vi "HEAD.vi"(0 "client handle":T4, 1 "Error code options":T2={"1xx (info)"=FALSE, "2xx (success)"=FALSE, "3xx (redirect)"=FALSE, "4xx (client error)"=TRUE, "5xx (server error)"=TRUE, "Other"=TRUE}, 2 "BlueLogParent in":refnum<class "BlueLogParent_OpenSource.lvclass">, 5 "url":string, 11 "error in (no error)":errorcluster, 12 "timeout (10000)":i32=10000) -> (4 "client handle out":T4, 6 "headers":T3[](array[typedef]), 10 "HTTP response code":T1, 15 "error out":errorcluster)   [LabVIEW 2020, in "Blue Easy HTTP OpenSource.lvlib"]
doc: "Sends a Web request that returns headers from a server, Web page, or Web service. This VI uses the HEAD HTTP method. This VI does not submit any data to the server or receive body data. The minimal data exchange makes the HEAD VI useful for testing the validity of a URL. Refer to the World Wide Web Consortium Web site at www.w3.org for more information about HTTP method definitions, including the HEAD method.\n\nYou can assign a client handle to add authentication credentials, HTTP headers, or a cookie to Web requests made by the HEAD VI. Use the OpenHandle VI to open a client handle and establish credentials. Use the AddHeader VI to add header lines to Web requests made by the HEAD VI."
uses:
  Blue Easy HTTP OpenSource.lvlib
  <vilib>/httpClient/ClientHandle.ctl
  HTTP Header.ctl
  HTTP error on codes.ctl
  HTTP response code.ctl
  <userlib>/Blue Origin/BlueLogParent_OpenSource/BlueLogParentClass/BlueLogParent_OpenSource.lvclass
  Interpret Header.vi
  <vilib>/dlg_ctls.llb/Space Constant.vi
  <vilib>/Utility/error.llb/Trim Whitespace.vi
  <vilib>/Utility/error.llb/Error Cluster From Error Code.vi
  <vilib>/httpClient/LabVIEWHTTPClient.lvlib
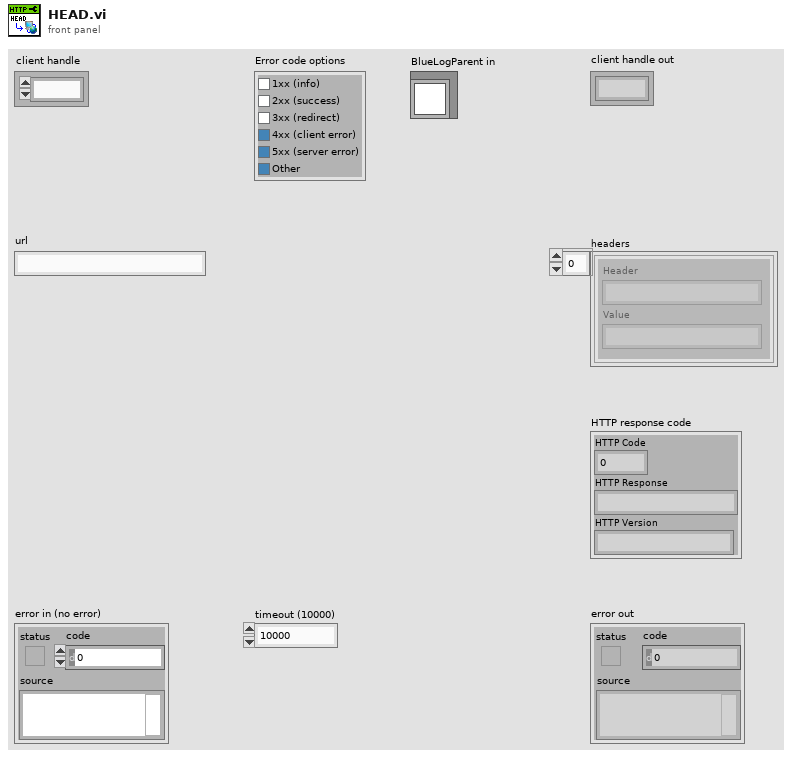
[diagram p1: front panel]
types:
  T1 = typedef "Blue Easy HTTP OpenSource.lvlib/HTTP response code.ctl" = cluster{"HTTP Code":u16, "HTTP Response":string, "HTTP Version":string}
  T2 = typedef "Blue Easy HTTP OpenSource.lvlib/HTTP error on codes.ctl" = cluster{"1xx (info)":bool, "2xx (success)":bool, "3xx (redirect)":bool, "4xx (client error)":bool, "5xx (server error)":bool, "Other":bool}
  T3 = typedef "Blue Easy HTTP OpenSource.lvlib/HTTP Header.ctl" = cluster{"Header":string, "Value":string}
  T4 = typedef "LabVIEWHTTPClient.lvlib/ClientHandle.ctl" = refnum<k1>
  T5 = typedef "BlueLogParent_OpenSource.lvclass/BlueLogParentLevel.ctl" = enum16{"DEBUG", "INFO", "WARNING", "ERROR", "CRITICAL"}
  T6 = typedef "BlueLogParent_OpenSource.lvclass/BlueLogParentOptions.ctl" = cluster{"timestamp (now)":dbl, "Call chain (here)":string, "Count (1)":u16, "Font (override)":T7, "Add row separator? (T)":bool}
  T7 = typedef "BlueLogParent_OpenSource.lvclass/BlueLogParentFont.ctl" = cluster{"Font Name":string, "Size":u16, "Bold":bool, "Italic":bool, "Underline":bool, "Strikeout":bool, "Color":u32}
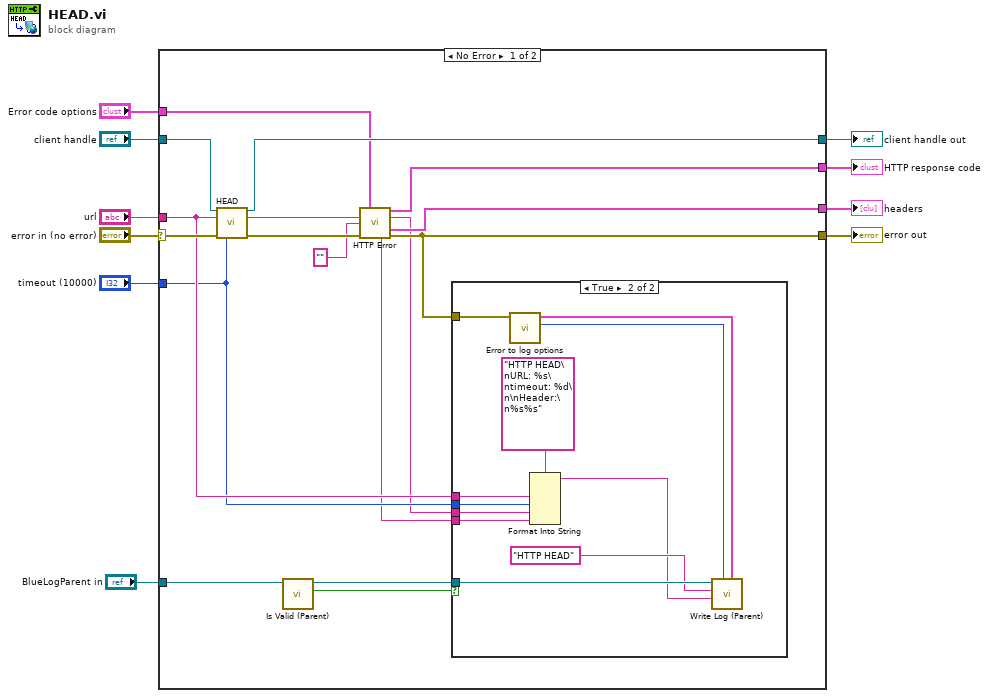
[diagram p0: block diagram]
diagram:
  n1 = case shown="No Error" "error in (no error)" {
    selector: "error in (no error)" -> [w27 w40]
    tunnel: [w16 w40] -> w10
    tunnel: "timeout (10000)" -> [w18 _]
    tunnel: "url" -> [w19 _]
    tunnel: "client handle" -> [w26 w39]
    tunnel: [w25 w39] -> w5
    tunnel: [w20 _] -> w4
    tunnel: "Error code options" -> [w23 _]
    tunnel: [w21 _] -> w2
    tunnel: "BlueLogParent in" -> [w15 _]
    frame No Error {
      n2 = call <vilib>:"HEAD.vi"("client handle"=w26, "url"=w19, "error in (no error)"=w27, "timeout (10000)"=w18) -> ("client handle out"=w25:T4, "headers"=w17:string, "error out"=w24:errorcluster)  [unwired: 9 in]
      n3 = call-dynamic "Is Valid (Parent).vi"("BlueLogParent in"=w15) -> ("Is Valid?"=w14:bool, "BlueLogParent out"=w13:refnum<class "BlueLogParent_OpenSource.lvclass">)  [unwired: 8 in, 1 out]
      n4 = call "HTTP Error.vi"("Error code options"=w23, "Header"=w17, "body"="", "error in (no error)"=w24) -> ("HTTP response code"=w21:T1, "Header (dup)"=w12:string, "Header Values"=w20:T3[], "Error log"=w11:string, "error out"=w16:errorcluster)  [unwired: 6 in, 1 out]
      n5 = case shown="True" w14 {
        tunnel: w16 -> [_ w33]
        tunnel: w19 -> [_ w37]
        tunnel: w12 -> [_ w36]
        tunnel: w18 -> [_ w35]
        tunnel: w13 -> [_ w34]
        tunnel: w11 -> [_ w28]
        frame False {
        }
        frame True {
          n6 = call "Error to log options.vi"("error in (no error)"=w33) -> ("Logging level"=w30:T5, "Options"=w29:T6)  [unwired: 9 in]
          n7 = Format Into String(format string="HTTP HEAD\nURL: %s\ntimeout: %d\n\nHeader:\n%s%s", w37, w35, w36, w28) -> (resulting string=w31:string)  [unwired: 2 in, 1 out]
          n8 = call-dynamic "Write Log (Parent).vi"("Options"=w29, "Logging level (INFO)"=w30, "Message"=w31, "Message Title"="HTTP HEAD" ("Unique ID"), "BlueLogParent in"=w34) -> ()  [unwired: 5 in, 2 out]
        }
      }
    }
    frame Error {
    }
  }
  "error out" <- w10
  "client handle out" <- w5
  "headers" <- w4
  "HTTP response code" <- w2
